vi "Simulation-02.vi"() -> (0 "lib error out":errorcluster, 3 "success":bool)   [LabVIEW 2020]
uses:
  librarian_class/typedefs/book_state--enum.ctl
  shared/request--enum.ctl
  librarian_class/librarian.lvclass
  client_class/client.lvclass
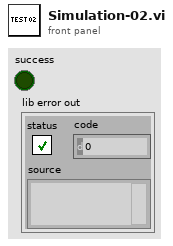
[diagram p1: front panel]
types:
  T1 = typedef "request--enum.ctl" = enum16{"CHECKIN", "CHECKOUT"}
  T2 = typedef "librarian.lvclass/book_state--enum.ctl" = enum16{"CHECKEDIN", "CHECKEDOUT", "DAMAGED"}
  T3 = typedef "message--cluster.ctl" = cluster{"header":string, "cmd":T1, "title":string, "book":string}
  T4 = typedef "librarian.lvclass/lib_map_value--cluster.ctl" = cluster{"book state":T2, "text":string, "hash":string}
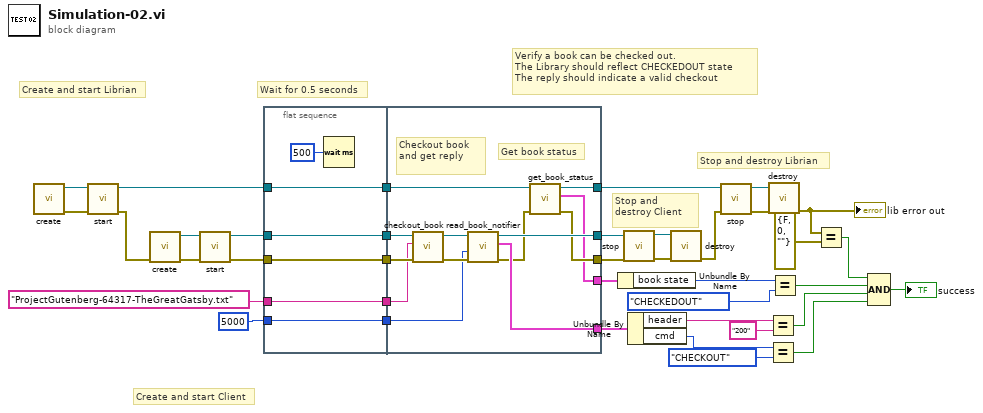
[diagram p0: block diagram]
diagram:
  # "Verify a book can be checked out.\nThe Library should reflect CHECKEDOUT state\nThe reply should indicate a valid checkout"
  # "Stop and destroy Client"
  # "Wait for 0.5 seconds"
  # "Create and start Client"
  # "Stop and destroy Librian"
  # "Create and start Librian"
  n1 = call "create.vi"() -> ("error out"=w37:errorcluster, "librarian_sm out"=w38:refnum<class "librarian.lvclass">)  [unwired: 10 in]
  n2 = call "start.vi"("error in (no error)"=w37, "librarian_sm in"=w38) -> ("error out"=w17:errorcluster, "librarian_sm out"=w28:refnum<class "librarian.lvclass">)  [unwired: 8 in]
  n3 = call "create.vi"("error in (no error)"=w17) -> ("error out"=w33:errorcluster, "librarian_sm out"=w34:refnum<class "client.lvclass">)  [unwired: 9 in]
  n4 = call "start.vi"("error in (no error)"=w33, "librarian_sm in"=w34) -> ("error out"=w30:errorcluster, "librarian_sm out"=w29:refnum<class "client.lvclass">)  [unwired: 8 in]
  n5 = flat-sequence {
    tunnel: "ProjectGutenberg-64317-TheGreatGatsby.txt" ("book title") -> [w40]
    tunnel: 5000 ("timeout in ms (-1)") -> [w42]
    tunnel: w28 -> [w43]
    tunnel: w29 -> [w44]
    tunnel: w30 -> [w39]
    tunnel: [w39] -> w22
    tunnel: [w44] -> w21
    tunnel: [w43] -> w20
    tunnel: [w42] -> w19
    tunnel: [w40] -> w18
    tunnel: [w48] -> w27
    tunnel: [w54] -> w26
    tunnel: [w46] -> w25
    tunnel: [w51] -> w14
    tunnel: w22 -> [w57]
    tunnel: w21 -> [w56]
    tunnel: w20 -> [w49]
    tunnel: w19 -> [w52]
    tunnel: w18 -> [w50]
    tunnel: [w45] -> w15
    frame #0 {
      n6 = Wait (ms)(milliseconds to wait=u32 500) -> ()  [unwired: 1 out]
    }
    frame #1 {
      # "Get book status"
      # "Checkout book and get reply"
      n7 = call "checkout_book.vi"("error in (no error)"=w57, "book title"=w50, "client in"=w56) -> ("error out"=w53:errorcluster, "client out"=w55:refnum<class "client.lvclass">)  [unwired: 7 in]
      n8 = call "read_book_notifier.vi"("error in (no error)"=w53, "timeout in ms (-1)"=w52, "client in"=w55) -> ("error out"=w47:errorcluster, "msg"=w51:T3, "client out"=w54:refnum<class "client.lvclass">)  [unwired: 6 in]
      n9 = call "get_book_status.vi"("error in (no error)"=w47, "librarian in"=w49) -> ("error out"=w46:errorcluster, "book status"=w45:T4, "librarian out"=w48:refnum<class "librarian.lvclass">)  [unwired: 7 in]
    }
  }
  n10 = Unbundle By Name(w15) -> ("book state"=w13:T2)
  n11 = call "stop.vi"("error in (no error)"=w25, "librarian_sm in"=w26) -> ("error out"=w31:errorcluster, "librarian_sm out"=w32:refnum<class "client.lvclass">)  [unwired: 8 in]
  n12 = Unbundle By Name(w14) -> ("header"=w11:string, "cmd"=w9:T1)
  n13 = call "destroy.vi"("error in (no error)"=w31, "librarian_sm in"=w32) -> ("error out"=w16:errorcluster)  [unwired: 8 in, 1 out]
  n14 = call "stop.vi"("error in (no error)"=w16, "librarian_sm in"=w27) -> ("error out"=w35:errorcluster, "librarian_sm out"=w36:refnum<class "librarian.lvclass">)  [unwired: 8 in]
  n15 = Equal?(x=w11, y="200") -> (x = y?=w3:bool)
  n16 = Equal?(x=w9, y=request--enum."CHECKOUT") -> (x = y?=w2:bool)
  n17 = call "destroy.vi"("error in (no error)"=w35, "librarian_sm in"=w36) -> ("error out"=w7:errorcluster)  [unwired: 8 in, 1 out]
  "lib error out" <- w7
  n18 = Equal?(x=w13, y=book_state--enum."CHECKEDOUT" ("book state")) -> (x = y?=w4:bool)
  n19 = Equal?(x=w7, y=errorcluster {"status"=FALSE, "code"=0, "source"=""}) -> (x = y?=w5:bool)
  n20 = Compound Arithmetic op=AND(w5, w4, w3, w2) -> (→"success":bool)
